vi "NamedNumericFactory.vi"(8 "error in":errorcluster, 11 "Gen Refnum":refnum<vi>) -> (0 "error out":errorcluster, 3 "NamedNumeric out":refnum<class "NamedNumeric.lvclass">)   [LabVIEW 2014, in "Raspberry Pi Compatible Compiler for LabVIEW.lvlib" / "NamedNumeric.lvclass"]
uses:
  NamedNumeric.lvclass
  Enum/Enum.lvclass
  Ring/Ring.lvclass
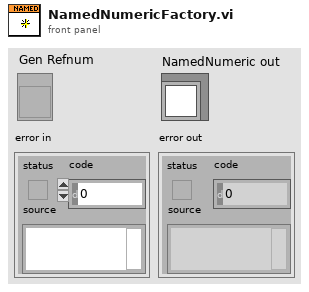
[diagram p1: front panel]
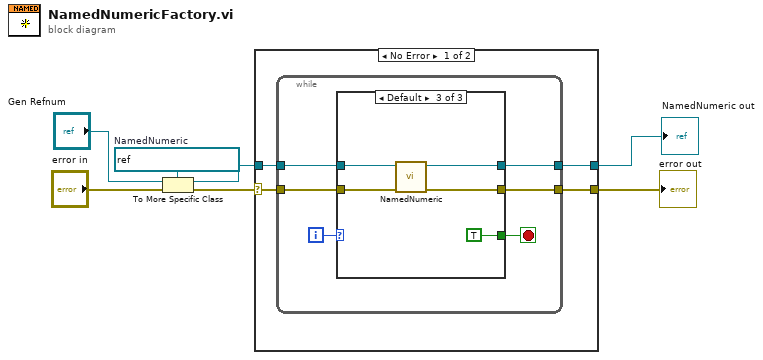
[diagram p0: block diagram]
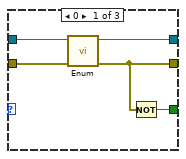
[diagram p2: hidden frame]
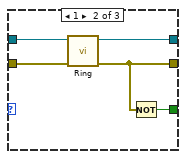
[diagram p3: hidden frame]
diagram:
  w6 = refnum<vi> refnum  # NamedNumeric
  n1 = To More Specific Class(target class=w6, reference="Gen Refnum", error in="error in") -> (specific class reference=w3:refnum<vi>, error out=w4:errorcluster)
  n2 = case shown="No Error" w4 {
    selector: w4 -> [w11 w33]
    tunnel: [w9 _] -> w1
    tunnel: [w8 w33] -> w2
    tunnel: w3 -> [w10 _]
    frame No Error {
      n3 = while {
        tunnel: w11 -> [w16]
        tunnel: [w15] -> w8
        tunnel: [w14] -> w9
        tunnel: w10 -> [w12]
        i -> [w17]
        stop <- w13 stop-if-true
        n4 = case shown="Default" w17 {
          tunnel: w16 -> [w22 w27 w30]
          tunnel: [w19 w24 w28] -> w15
          tunnel: [w21 w26 w29] -> w14
          tunnel: [w20 w25 TRUE] -> w13
          tunnel: w12 -> [w18 w23 w31]
          frame 0 {
            n5 = call "Enum.vi"("error in"=w22, "GObj Refnum"=w18) -> ("error out"=w19:errorcluster, "Enum out"=w21:refnum<class "Enum.lvclass">)  [unwired: 8 in]
            n6 = Not(x=w19) -> (.not. x?=w20:bool)
          }
          frame 1 {
            n7 = call "Ring.vi"("error in"=w27, "GObj Refnum"=w23) -> ("error out"=w24:errorcluster, "Ring out"=w26:refnum<class "Ring.lvclass">)  [unwired: 8 in]
            n8 = Not(x=w24) -> (.not. x?=w25:bool)
          }
          frame Default {
            n9 = call "NamedNumeric.vi"("error in"=w30, "GObj Refnum"=w31) -> ("error out"=w28:errorcluster, "Digital out"=w29:refnum<class "NamedNumeric.lvclass">)  [unwired: 8 in]
          }
        }
      }
    }
    frame Error {
    }
  }
  "error out" <- w2
  "NamedNumeric out" <- w1
